vi "MulColLBTable-Array-OPs.vi"(0 "MulColLBTable-Array.lvclass IN":refnum<class "MulColLBTable-Array.lvclass">, 1 "Multi-col LB Refs":refnum<vi>[](array[refnum]), 2 "Operations":T1, 5 "Item Names - Bulk / stack Multiple":string[][][](array[string]), 7 "Item Names - stack single":string[][](array[string]), 9 "Value":i32[][](array[numeric]), 11 "error in (no error)":errorcluster, 12 "Column Header Strings[]":string[][](array[string])) -> (4 "MulColLBTable-Array.lvclass OUT":refnum<class "MulColLBTable-Array.lvclass">, 15 "error out":errorcluster)   [LabVIEW 2020, in "MulColLBTable-Array.lvclass"]
uses:
  MulColLBTable-Array.lvclass
  Object operations.ctl
  MulColLBTable-Array.lvclass/MulColLBTable-Array.ctl
  MulColLBTable/MulColLBTable.lvclass
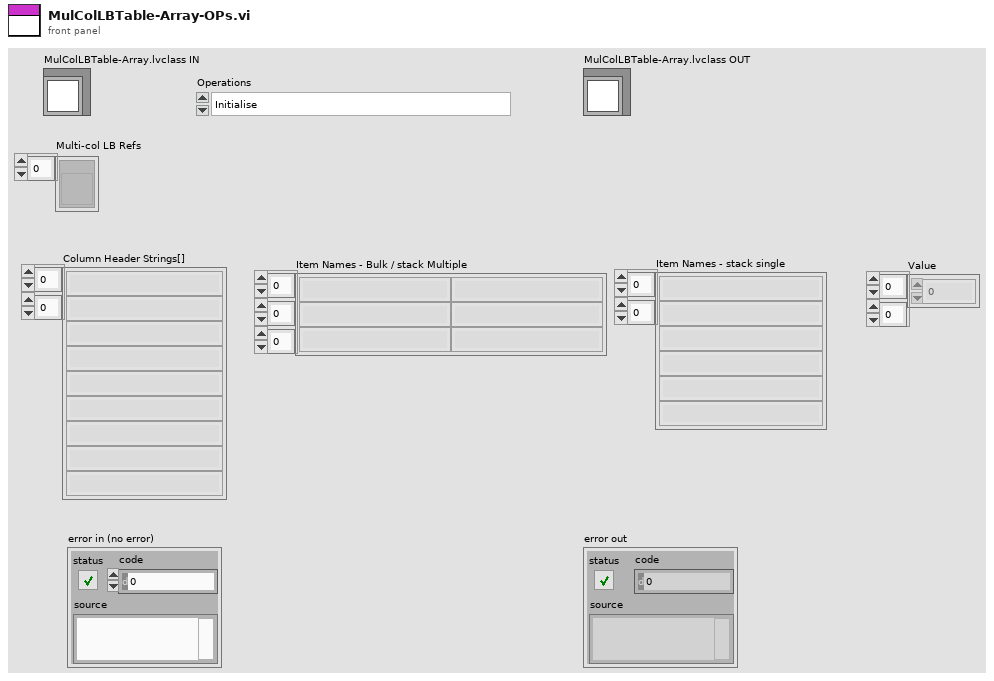
[diagram p1: front panel]
types:
  T1 = typedef "Object operations.ctl" = enum16{"Initialise", "Add column headers", "Add rows - bulk", "Stack row - single", "Stack row - multi", "Select row(s)", "Delete row(s)", "Destroy"}
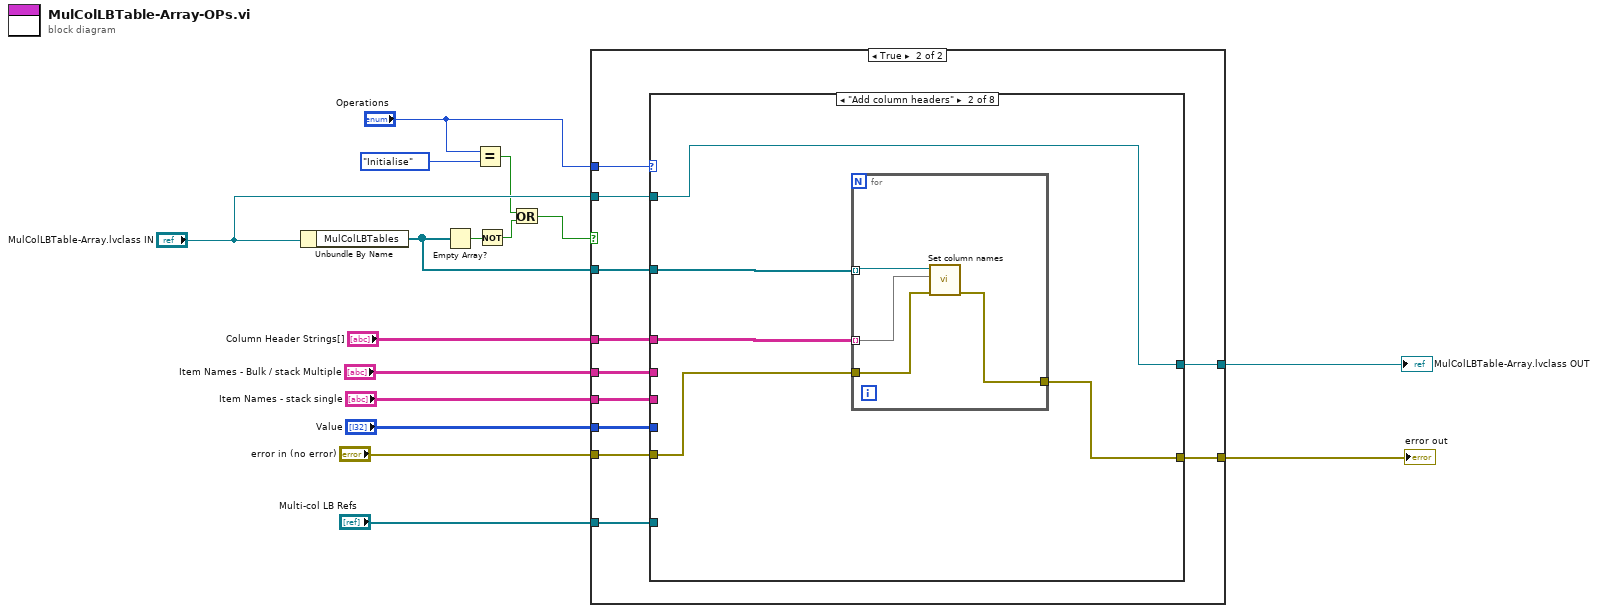
[diagram p0: block diagram]
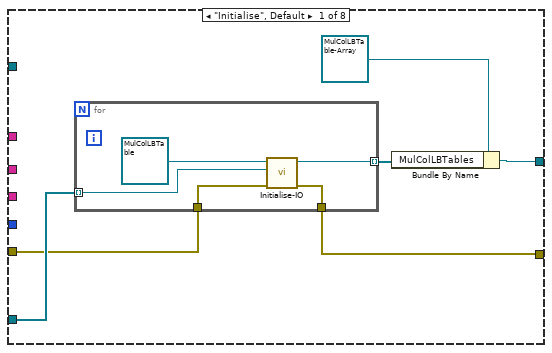
[diagram p3: hidden frame]
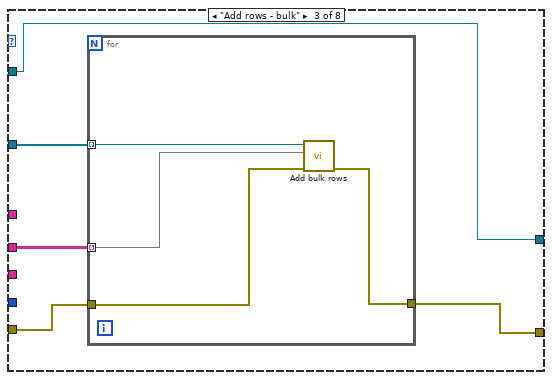
[diagram p4: hidden frame]
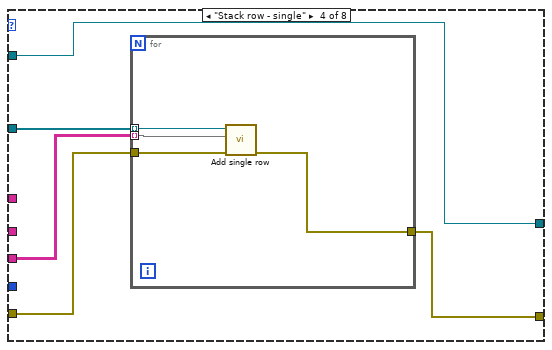
[diagram p5: hidden frame]
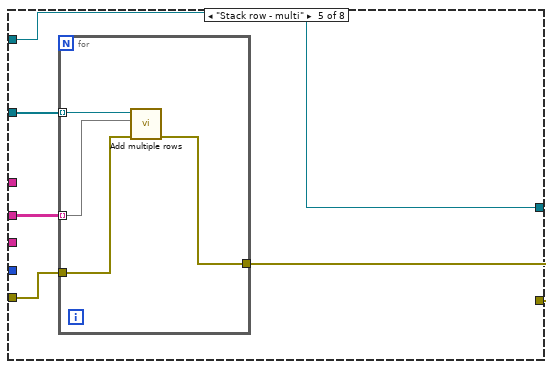
[diagram p6: hidden frame]
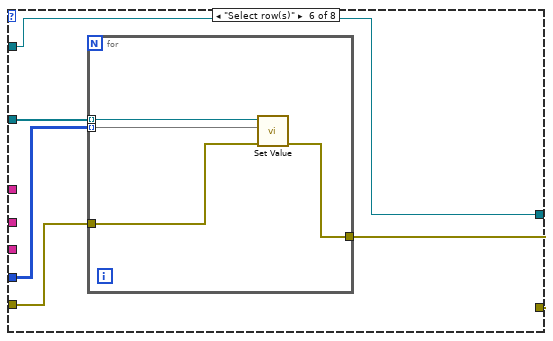
[diagram p7: hidden frame]
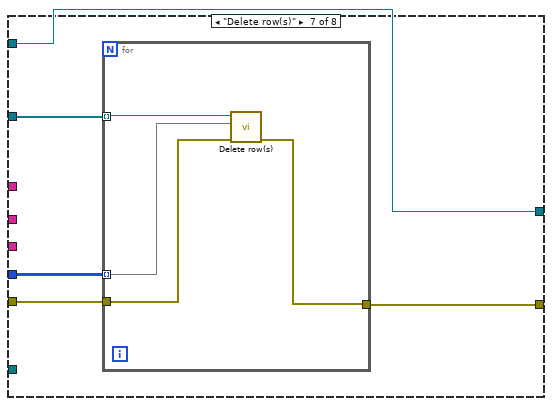
[diagram p8: hidden frame]
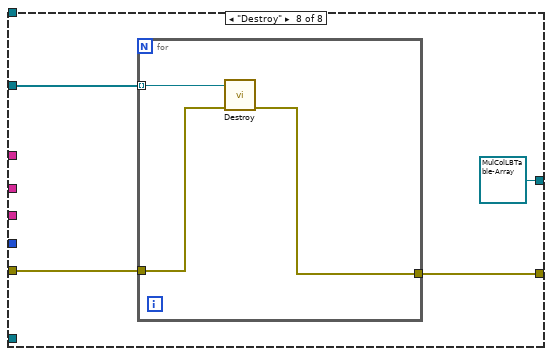
[diagram p9: hidden frame]
diagram:
  n1 = Unbundle By Name("MulColLBTable-Array.lvclass IN") -> ("MulColLBTables"=w7:refnum<class "MulColLBTable.lvclass">[])
  n2 = Empty Array?(array=w7) -> (empty?=w6:bool)
  n3 = Equal?(x="Operations", y=Object_operations."Initialise") -> (x = y?=w2:bool)
  n4 = Not(x=w6) -> (.not. x?=w5:bool)
  n5 = Or(x=w2, y=w5) -> (x .or. y?=w1:bool)
  n6 = case shown="True" w1 {
    tunnel: "Multi-col LB Refs" -> [_ w29]
    tunnel: "error in (no error)" -> [w17 w28]
    tunnel: [w17 w27] -> w14
    tunnel: "Operations" -> [_ w26]
    tunnel: w7 -> [_ w25]
    tunnel: "Column Header Strings[]" -> [_ w24]
    tunnel: "Item Names - Bulk / stack Multiple" -> [_ w23]
    tunnel: "Item Names - stack single" -> [_ w22]
    tunnel: [w18 w21] -> w10
    tunnel: "MulColLBTable-Array.lvclass IN" -> [w18 w20]
    tunnel: "Value" -> [_ w19]
    frame False {
    }
    frame True {
      n7 = case shown="\"Add column headers\"" w26 {
        tunnel: w29 -> [w33 _ _ _ _ _ _ _]
        tunnel: w28 -> [w32 w45 w51 w61 w69 w78 w87 w96]
        tunnel: [w31 w44 w50 w60 w68 w77 w86 w95] -> w27
        tunnel: w25 -> [_ w43 w54 w63 w72 w81 w90 w98]
        tunnel: w24 -> [_ w42 _ _ _ _ _ _]
        tunnel: w23 -> [_ _ w53 _ w70 _ _ _]
        tunnel: w22 -> [_ _ _ w62 _ _ _ _]
        tunnel: [w30 w41 w52 w59 w71 w79 w88 refnum<class "MulColLBTable-Array.lvclass"> refnum ("MulColLBTable-Array.lvclass IN")] -> w21
        tunnel: w20 -> [_ w41 w52 w59 w71 w79 w88 _]
        tunnel: w19 -> [_ _ _ _ _ w80 w89 _]
        frame "Initialise", Default {
          n8 = for {
            tunnel: [w40] -> w34 mode=indexing
            tunnel: w33 -> [w36] mode=indexing
            tunnel: w32 -> [w38]
            tunnel: [w37] -> w31
            n9 = call "Initialise-IO.vi"("error in (no error)"=w38, "Multicolumn Listbox"=w36, "MulColLBTable.lvclass"=refnum<class "MulColLBTable.lvclass"> refnum) -> ("error out"=w37:errorcluster, "MulColLBTable.lvclass out"=w40:refnum<class "MulColLBTable.lvclass">)  [unwired: 7 in]
          }
          n10 = Bundle By Name(cluster=refnum<class "MulColLBTable-Array.lvclass"> refnum ("MulColLBTable-Array.lvclass"), "MulColLBTables"=w34) -> (w30:refnum<class "MulColLBTable-Array.lvclass">)
        }
        frame "Add column headers" {
          n11 = for {
            tunnel: w43 -> [w49] mode=indexing
            tunnel: w42 -> [w48] mode=indexing
            tunnel: w45 -> [w47]
            tunnel: [w46] -> w44
            n12 = call "Set column names.vi"("error in (no error)"=w47, "Column Header Strings[]"=w48, "MulColLBTable.lvclass"=w49) -> ("error out"=w46:errorcluster)  [unwired: 7 in, 1 out]
          }
        }
        frame "Add rows - bulk" {
          n13 = for {
            tunnel: w54 -> [w58] mode=indexing
            tunnel: w53 -> [w57] mode=indexing
            tunnel: w51 -> [w56]
            tunnel: [w55] -> w50
            n14 = call "Add bulk rows.vi"("error in (no error)"=w56, "Item Names"=w57, "MulColLBTable.lvclass"=w58) -> ("error out"=w55:errorcluster)  [unwired: 7 in, 1 out]
          }
        }
        frame "Stack row - single" {
          n15 = for {
            tunnel: w63 -> [w67] mode=indexing
            tunnel: w62 -> [w66] mode=indexing
            tunnel: w61 -> [w65]
            tunnel: [w64] -> w60
            n16 = call "Add single row.vi"("error in (no error)"=w65, "Row"=w66, "MulColLBTable.lvclass"=w67) -> ("error out"=w64:errorcluster)  [unwired: 7 in, 1 out]
          }
        }
        frame "Stack row - multi" {
          n17 = for {
            tunnel: w72 -> [w76] mode=indexing
            tunnel: w70 -> [w75] mode=indexing
            tunnel: w69 -> [w74]
            tunnel: [w73] -> w68
            n18 = call "Add multiple rows.vi"("error in (no error)"=w74, "Row"=w75, "MulColLBTable.lvclass"=w76) -> ("error out"=w73:errorcluster)  [unwired: 7 in, 1 out]
          }
        }
        frame "Select row(s)" {
          n19 = for {
            tunnel: w81 -> [w85] mode=indexing
            tunnel: w80 -> [w84] mode=indexing
            tunnel: w78 -> [w83]
            tunnel: [w82] -> w77
            n20 = call "Set Value.vi"("error in (no error)"=w83, "Value"=w84, "MulColLBTable.lvclass"=w85) -> ("error out"=w82:errorcluster)  [unwired: 7 in, 1 out]
          }
        }
        frame "Delete row(s)" {
          n21 = for {
            tunnel: w90 -> [w94] mode=indexing
            tunnel: w89 -> [w93] mode=indexing
            tunnel: w87 -> [w92]
            tunnel: [w91] -> w86
            n22 = call "Delete row(s).vi"("error in (no error)"=w92, "Row Indices"=w93, "MulColLBTable.lvclass"=w94) -> ("error out"=w91:errorcluster)  [unwired: 7 in, 1 out]
          }
        }
        frame "Destroy" {
          n23 = for {
            tunnel: w98 -> [w101] mode=indexing
            tunnel: w96 -> [w100]
            tunnel: [w99] -> w95
            n24 = call "Destroy.vi"("error in (no error)"=w100, "MulColLBTable.lvclass"=w101) -> ("error out"=w99:errorcluster)  [unwired: 9 in]
          }
        }
      }
    }
  }
  "MulColLBTable-Array.lvclass OUT" <- w10
  "error out" <- w14
